vi "Finish.vi"   [LabVIEW 2012]
doc: "This VI is called just before exiting. It is expected to close I/O refnum, save collected data, etc."
uses:
  Begin/Global Refnums.vi
  <vilib>/Rock Robotics/WPI/RobotDrive/WPI_RobotDriveGetSetRefNum.vi
  <vilib>/Rock Robotics/WPI/Joystick/WPI_JoystickGetSetRefNum.vi
types:
  T1 = typedef "WPI_RobotDriveDevRef.ctl" = cluster{"DevStatus":errorcluster, "Motors[]":T2[], "Square Inputs":bool, "Max Output":dbl, "Isochronous":bool}
  T2 = typedef "WPI_MotorControlDeviceRef.ctl" = cluster{"DeviceStatus":errorcluster, "Type":enum16{"PWM", "CAN"}, "PWM":cluster{"Digital Module":T3, "PWM Channel":T4, "DeadBand":T5}, "CAN":cluster{"Device Number":u8, "Control Mode":T6, "Semaphore":T7, "Max Vout":dbl}, "Invert":bool, "TransformRef":T8, "InvTransformRef":T8}
  T3 = typedef "FPGA_TypedefDigitalModule.ctl" = enum16{"Digital Module 1", "Digital Module 2"}
  T4 = typedef "FPGA_DIOPWMChannel.ctl" = enum8{"PWM 1", "PWM 2", "PWM 3", "PWM 4", "PWM 5", "PWM 6", "PWM 7", "PWM 8", "PWM 9", "PWM 10", "Invalid"}
  T5 = typedef "WPI_PWMDeadband.ctl" = cluster{"Name":string, "maxPositivePwm":i32, "minPositivePwm":i32, "centerPwm":i32, "maxNegativePwm":i32, "minNegativePwm":i32, "angularRange":u16}
  T6 = typedef "WPI_CANJaguar_ControlMode.ctl" = enum8{"Percent VBus", "Current", "Speed", "Position", "Voltage"}
  T7 = typedef "Semaphore RefNum" = refnum<k1>
  T8 = typedef "WPI_PWMTransform_ConPane.ctl" = refnum<vi>
  T9 = typedef "WPI_JoystickDevRef.ctl" = cluster{"Device":T10}
  T10 = typedef "WPI_JoystickDeviceEnum.ctl" = enum16{"USB 1", "USB 2", "USB 3", "USB 4", "Kinect 1", "Kinect 2"}
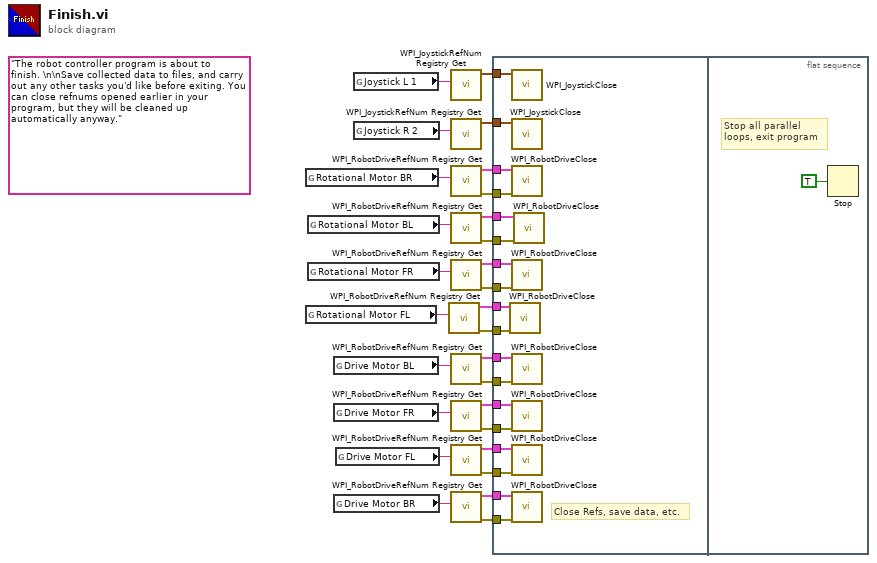
[diagram p0: block diagram]
diagram:
  (unwired) "The robot controller program is about to finish. \n\nSave collected data to files, and carry out any other tasks you'd like before exiting. You can close refnums opened earlier in your program, but they will be cleaned up automatically anyway."
  n1 = global read "Global Refnums.vi" "Rotational Motor BR"() -> (w7:string)
  n2 = global read "Global Refnums.vi" "Rotational Motor FL"() -> (w6:string)
  n3 = global read "Global Refnums.vi" "Rotational Motor BL"() -> (w8:string)
  n4 = global read "Global Refnums.vi" "Rotational Motor FR"() -> (w5:string)
  n5 = global read "Global Refnums.vi" "Drive Motor BL"() -> (w4:string)
  n6 = global read "Global Refnums.vi" "Drive Motor FR"() -> (w1:string)
  n7 = global read "Global Refnums.vi" "Drive Motor BR"() -> (w3:string)
  n8 = global read "Global Refnums.vi" "Drive Motor FL"() -> (w2:string)
  n9 = global read "Global Refnums.vi" "Joystick L 1"() -> (w25:string)
  n10 = global read "Global Refnums.vi" "Joystick R 2"() -> (w24:string)
  n11 = call <vilib>:"WPI_RobotDriveRefNum Registry Get.vi"("refnum name"=w6) -> ("error out"=w13:errorcluster, "RobotDriveDevRef"=w14:T1)  [unwired: 1 in, 8 out]
  n12 = call <vilib>:"WPI_JoystickRefNum Registry Get.vi"("refnum name"=w25) -> ("JoystickDevRef"=w27:T9)  [unwired: 1 in, 9 out]
  n13 = call <vilib>:"WPI_JoystickRefNum Registry Get.vi"("refnum name"=w24) -> ("JoystickDevRef"=w26:T9)  [unwired: 1 in, 9 out]
  n14 = call <vilib>:"WPI_RobotDriveRefNum Registry Get.vi"("refnum name"=w7) -> ("error out"=w11:errorcluster, "RobotDriveDevRef"=w12:T1)  [unwired: 1 in, 8 out]
  n15 = call <vilib>:"WPI_RobotDriveRefNum Registry Get.vi"("refnum name"=w8) -> ("error out"=w9:errorcluster, "RobotDriveDevRef"=w10:T1)  [unwired: 1 in, 8 out]
  n16 = call <vilib>:"WPI_RobotDriveRefNum Registry Get.vi"("refnum name"=w5) -> ("error out"=w17:errorcluster, "RobotDriveDevRef"=w16:T1)  [unwired: 1 in, 8 out]
  n17 = call <vilib>:"WPI_RobotDriveRefNum Registry Get.vi"("refnum name"=w4) -> ("error out"=w18:errorcluster, "RobotDriveDevRef"=w15:T1)  [unwired: 1 in, 8 out]
  n18 = call <vilib>:"WPI_RobotDriveRefNum Registry Get.vi"("refnum name"=w1) -> ("error out"=w19:errorcluster, "RobotDriveDevRef"=w28:T1)  [unwired: 1 in, 8 out]
  n19 = call <vilib>:"WPI_RobotDriveRefNum Registry Get.vi"("refnum name"=w2) -> ("error out"=w20:errorcluster, "RobotDriveDevRef"=w23:T1)  [unwired: 1 in, 8 out]
  n20 = call <vilib>:"WPI_RobotDriveRefNum Registry Get.vi"("refnum name"=w3) -> ("error out"=w21:errorcluster, "RobotDriveDevRef"=w22:T1)  [unwired: 1 in, 8 out]
  n21 = flat-sequence {
    tunnel: w28 -> [w46]
    tunnel: w27 -> [w45]
    tunnel: w26 -> [w44]
    tunnel: w23 -> [w43]
    tunnel: w22 -> [w42]
    tunnel: w21 -> [w41]
    tunnel: w20 -> [w40]
    tunnel: w19 -> [w39]
    tunnel: w18 -> [w38]
    tunnel: w17 -> [w37]
    tunnel: w16 -> [w36]
    tunnel: w15 -> [w35]
    tunnel: w14 -> [w34]
    tunnel: w13 -> [w33]
    tunnel: w12 -> [w32]
    tunnel: w11 -> [w31]
    tunnel: w10 -> [w30]
    tunnel: w9 -> [w29]
    frame #0 {
      # "Close Refs, save data, etc."
      n22 = call <vilib>:"WPI_RobotDriveClose.vi"("error in (no error)"=w33, "RobotDriveDevRef"=w34) -> ()  [unwired: 10 out]
      n23 = call <vilib>:"WPI_JoystickClose.vi"("JoystickDevRef"=w45) -> ()  [unwired: 11 out]
      n24 = call <vilib>:"WPI_JoystickClose.vi"("JoystickDevRef"=w44) -> ()  [unwired: 11 out]
      n25 = call <vilib>:"WPI_RobotDriveClose.vi"("error in (no error)"=w31, "RobotDriveDevRef"=w32) -> ()  [unwired: 10 out]
      n26 = call <vilib>:"WPI_RobotDriveClose.vi"("error in (no error)"=w37, "RobotDriveDevRef"=w36) -> ()  [unwired: 10 out]
      n27 = call <vilib>:"WPI_RobotDriveClose.vi"("error in (no error)"=w38, "RobotDriveDevRef"=w35) -> ()  [unwired: 10 out]
      n28 = call <vilib>:"WPI_RobotDriveClose.vi"("error in (no error)"=w39, "RobotDriveDevRef"=w46) -> ()  [unwired: 10 out]
      n29 = call <vilib>:"WPI_RobotDriveClose.vi"("error in (no error)"=w40, "RobotDriveDevRef"=w43) -> ()  [unwired: 10 out]
      n30 = call <vilib>:"WPI_RobotDriveClose.vi"("error in (no error)"=w41, "RobotDriveDevRef"=w42) -> ()  [unwired: 10 out]
      n31 = call <vilib>:"WPI_RobotDriveClose.vi"("error in (no error)"=w29, "RobotDriveDevRef"=w30) -> ()  [unwired: 10 out]
    }
    frame #1 {
      # "Stop all parallel\nloops, exit program"
      n32 = Stop(stop? (T)=TRUE ("Quit")) -> ()
    }
  }
